vi "Plot Sine Graph x0.vi"() -> ()   [LabVIEW 2020]
panel:
  out "Data":dbl[](array[numeric])
  out "Waveform Graph":cluster{i32, i32, dbl[]}(graph)
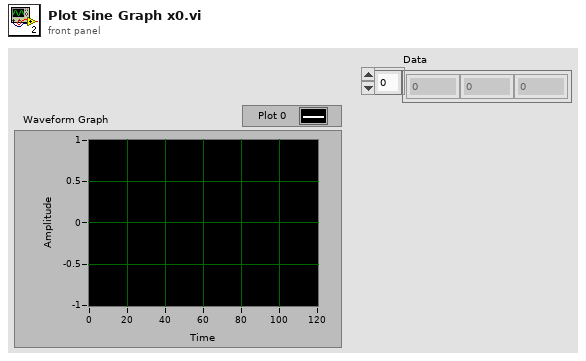
[diagram p1: front panel]
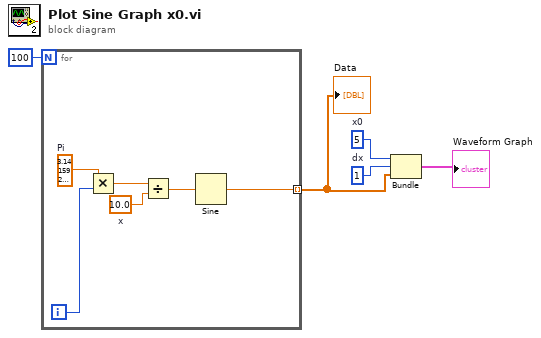
[diagram p0: block diagram]
diagram:
  w3 = 1  # dx
  w4 = 5  # x0
  n1 = for {
    N: 100 -> [_]
    tunnel: [w6] -> w2 mode=indexing
    i -> [w11]
    w8 = 10.0  # x
    w10 = 3.141592653589793  # Pi
    n2 = Multiply(x=w10, y=w11) -> (x*y=w9:dbl)
    n3 = Divide(x=w9, y=w8) -> (x/y=w7:dbl)
    n4 = Sine(x=w7) -> (sin(x)=w6:dbl)
  }
  "Data" <- w2
  n5 = Bundle "Bundle"("x0"=w4, "dx"=w3, w2) -> (→"Waveform Graph":cluster{"x0":i32, "dx":i32, dbl[]})  [unwired: 1 in]
